vi "varrange.vi"() -> ()   [LabVIEW 2012]
panel:
  out "range":i32
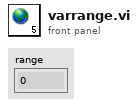
[diagram p1: front panel]
diagram:
